vi "Draw_Line.vi"(6 "light?":bool=TRUE, 8 "Draw?":bool=TRUE, 9 "end":cluster{"x":dbl, "y":dbl}, 10 "start":cluster{"x":dbl, "y":dbl}, 11 "picture in":picture) -> (1 "line":cluster{"slope":dbl, "b":dbl, "theta":dbl}, 3 "picture out":picture)   [LabVIEW 2022 SP3]
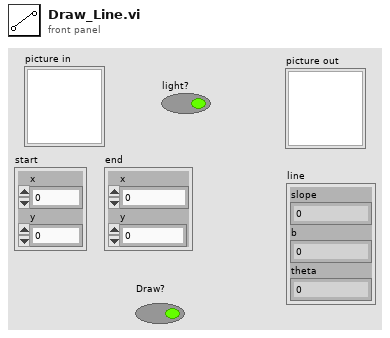
[diagram p1: front panel]
types:
  T1 = cluster{"Width":u16, "Style":enum32{"Solid", "Dash", "Dot", "DashDot", "DashDotDot"}}
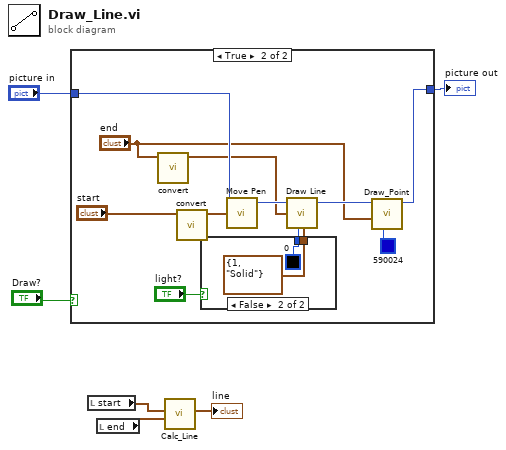
[diagram p0: block diagram]
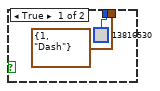
[diagram p3: hidden frame]
diagram:
  n1 = case shown="True" "Draw?" {
    tunnel: "picture in" -> [w7 w17]
    tunnel: [w7 w8] -> w2
    frame False {
    }
    frame True {
      n2 = call "convert.vi"("point"="end") -> ("scaled"=w12:cluster{"x":dbl, "y":dbl})  [unwired: 10 in]
      n3 = call "convert.vi"("point"="start") -> ("scaled"=w13:cluster{"x":dbl, "y":dbl})  [unwired: 10 in]
      n4 = case shown="False" "light?" {
        tunnel: [u32 13816530 ("color(black)") u32 0 ("color(black)")] -> w19
        tunnel: [T1 {"Width"=1, "Style"=enum."Dash"} ("pen") T1 {"Width"=1, "Style"=enum."Solid"} ("pen")] -> w18
        frame True {
        }
        frame False {
        }
      }
      n5 = call <vilib>:"Move Pen.vi"("new position"=w13, "picture"=w17) -> ("new picture"=w16:picture)  [unwired: 3 in]
      n6 = call <vilib>:"Draw Line.vi"("picture"=w16, "end point"=w12, "color(black)"=w19, "pen"=w18) -> ("new picture"=w11:picture)  [unwired: 5 in]
      n7 = call "Draw_Point.vi"("color"=u32 590024 ("color(black)"), "point"="end", "picture in"=w11) -> ("new picture"=w8:picture)  [unwired: 8 in]
    }
  }
  "picture out" <- w2
  n8 = local read "start"() -> (w5:cluster{"x":dbl, "y":dbl})
  n9 = local read "end"() -> (w4:cluster{"x":dbl, "y":dbl})
  n10 = call "Calc_Line.vi"("end"=w4, "start"=w5) -> ("line"=→"line":cluster{"slope":dbl, "b":dbl, "theta":dbl})  [unwired: 9 in]
